vi "08Foot.vi"() -> ()   [LabVIEW 2015]
uses:
  <vilib>/Instr/_visa.llb/VISA Configure Serial Port (Serial Instr).vi
  <vilib>/Utility/file.llb/Read Delimited Spreadsheet (DBL).vi
  <vilib>/DAQmx/create/channels.llb/DAQmx Create Channel (DI-Digital Input).vi
  <vilib>/DAQmx/configure/timing.llb/DAQmx Timing (Sample Clock).vi
  <vilib>/Utility/file.llb/Write Delimited Spreadsheet (DBL).vi
  <resource>/objmgr/daqmx.rc
panel:
  in  "Tab Control":enum32{"Page 1", "Page 2"}(tab)
  out "NEXT MPH 2":dbl min=0.0 max=12.0 step=0.1 format="%.2f"
  out "MPH 2":dbl min=0.0 max=12.0 step=0.1 format="%.2f"
  out "NEXT DURATION":dbl format="%#.1f"
  out "Time Left":dbl format="%#.0f"
  out "ESTOP":bool
  in  "ESTOP RESUME":bool
  out "MPH READ":u8
  out "Foot":dbl
  out "ESTOP2":bool
  out "Report Location":path
  in  "TestScript":path=path "C:/LabVIEW VIs/TRMConsole/FootTime.txt"
  out "Waveform Graph":dbl[](graph)
  out "speed":dbl[](array[numeric])
  out "time":dbl[](array[numeric])
  out "dwell":dbl[](array[numeric])
  out "step":i32
  out "arraysize":i32
  out "x-y":u32
  out "appended path":path
  out "stopping":bool
  out "String":string
  in  "stop":bool
  in  "Serial Port":refnum<visa-resource-name>="COM8"
  in  "lines":tag="DAQMod1/port0"
  out "Enum":T1(ring)
  out "NEXT MPH":dbl min=0.0 max=12.0 step=0.1 format="%.1f"
  out "MPH":dbl min=0.0 max=12.0 step=0.1 format="%.1f"
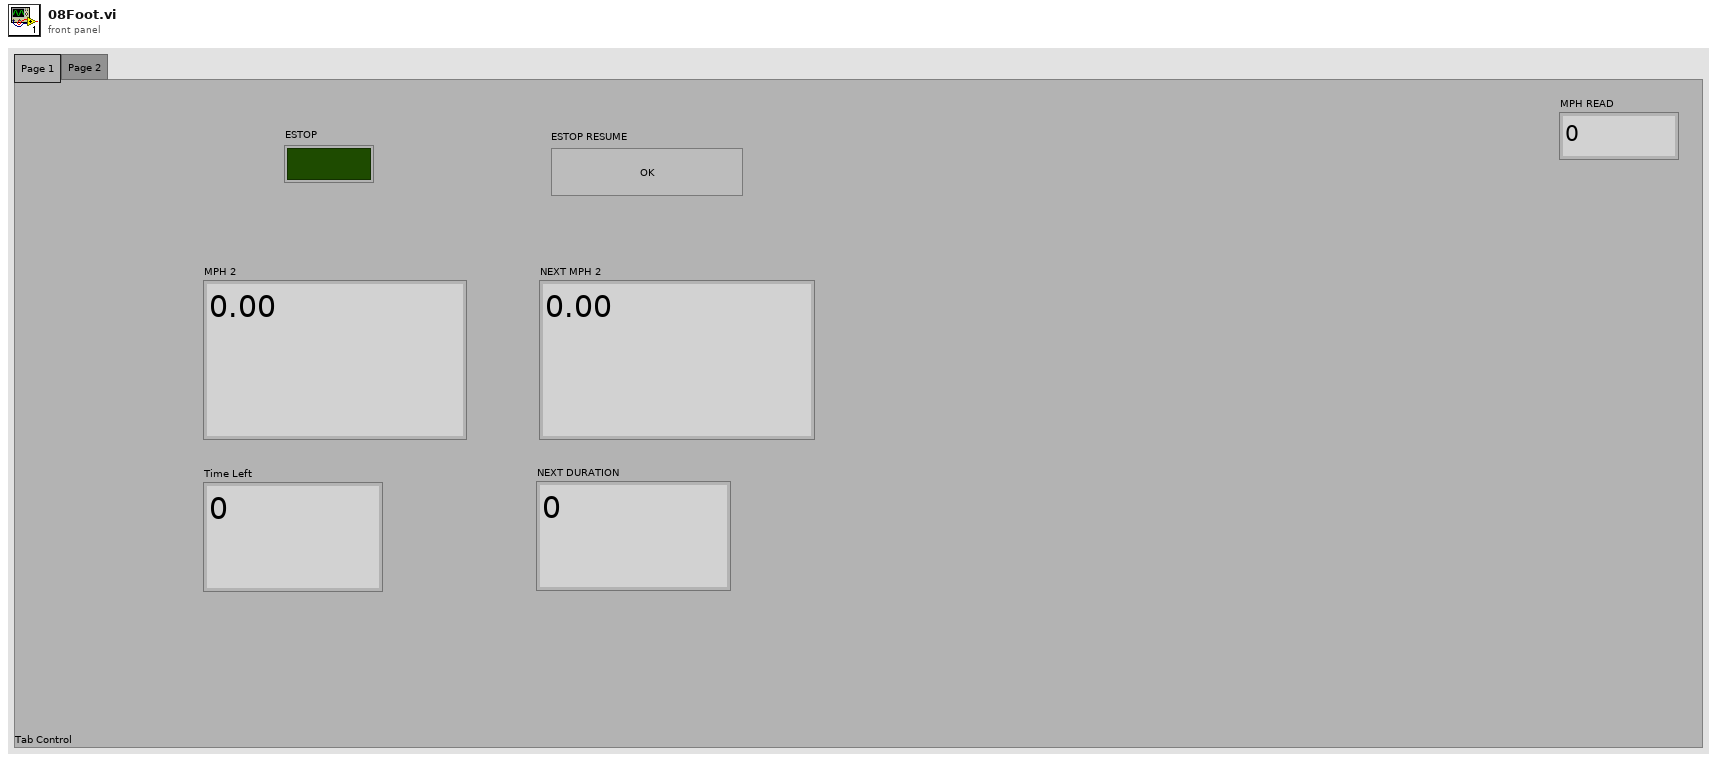
[diagram p1: front panel]
types:
  T1 = enum16{"Initialize", "SetMPH", "GetData", "CheckTiming", "CompressWave", "StartDAQ", "StopDAQ", "Dwell", "WaitforMPH", "ESTOP Wait", "ESTOP Resume"}
  T2 = enum16{"Initialize", "SetMPH", "GetData", "CheckTiming", "CompressWave", "StartDAQ", "StopDAQ", "Dwell", "WaitforMPH"}
  T3 = enum16{"Initialize", "SetMPH", "GetData", "CheckTiming", "CompressWave", "StartDAQ"}
  T4 = enum16{"Initialize", "SetMPH", "GetData", "CheckTiming", "CompressWave"}
  T5 = enum16{"Initialize", "SetMPH", "GetData", "CheckTiming", "CompressWave", "StartDAQ", "StopDAQ"}
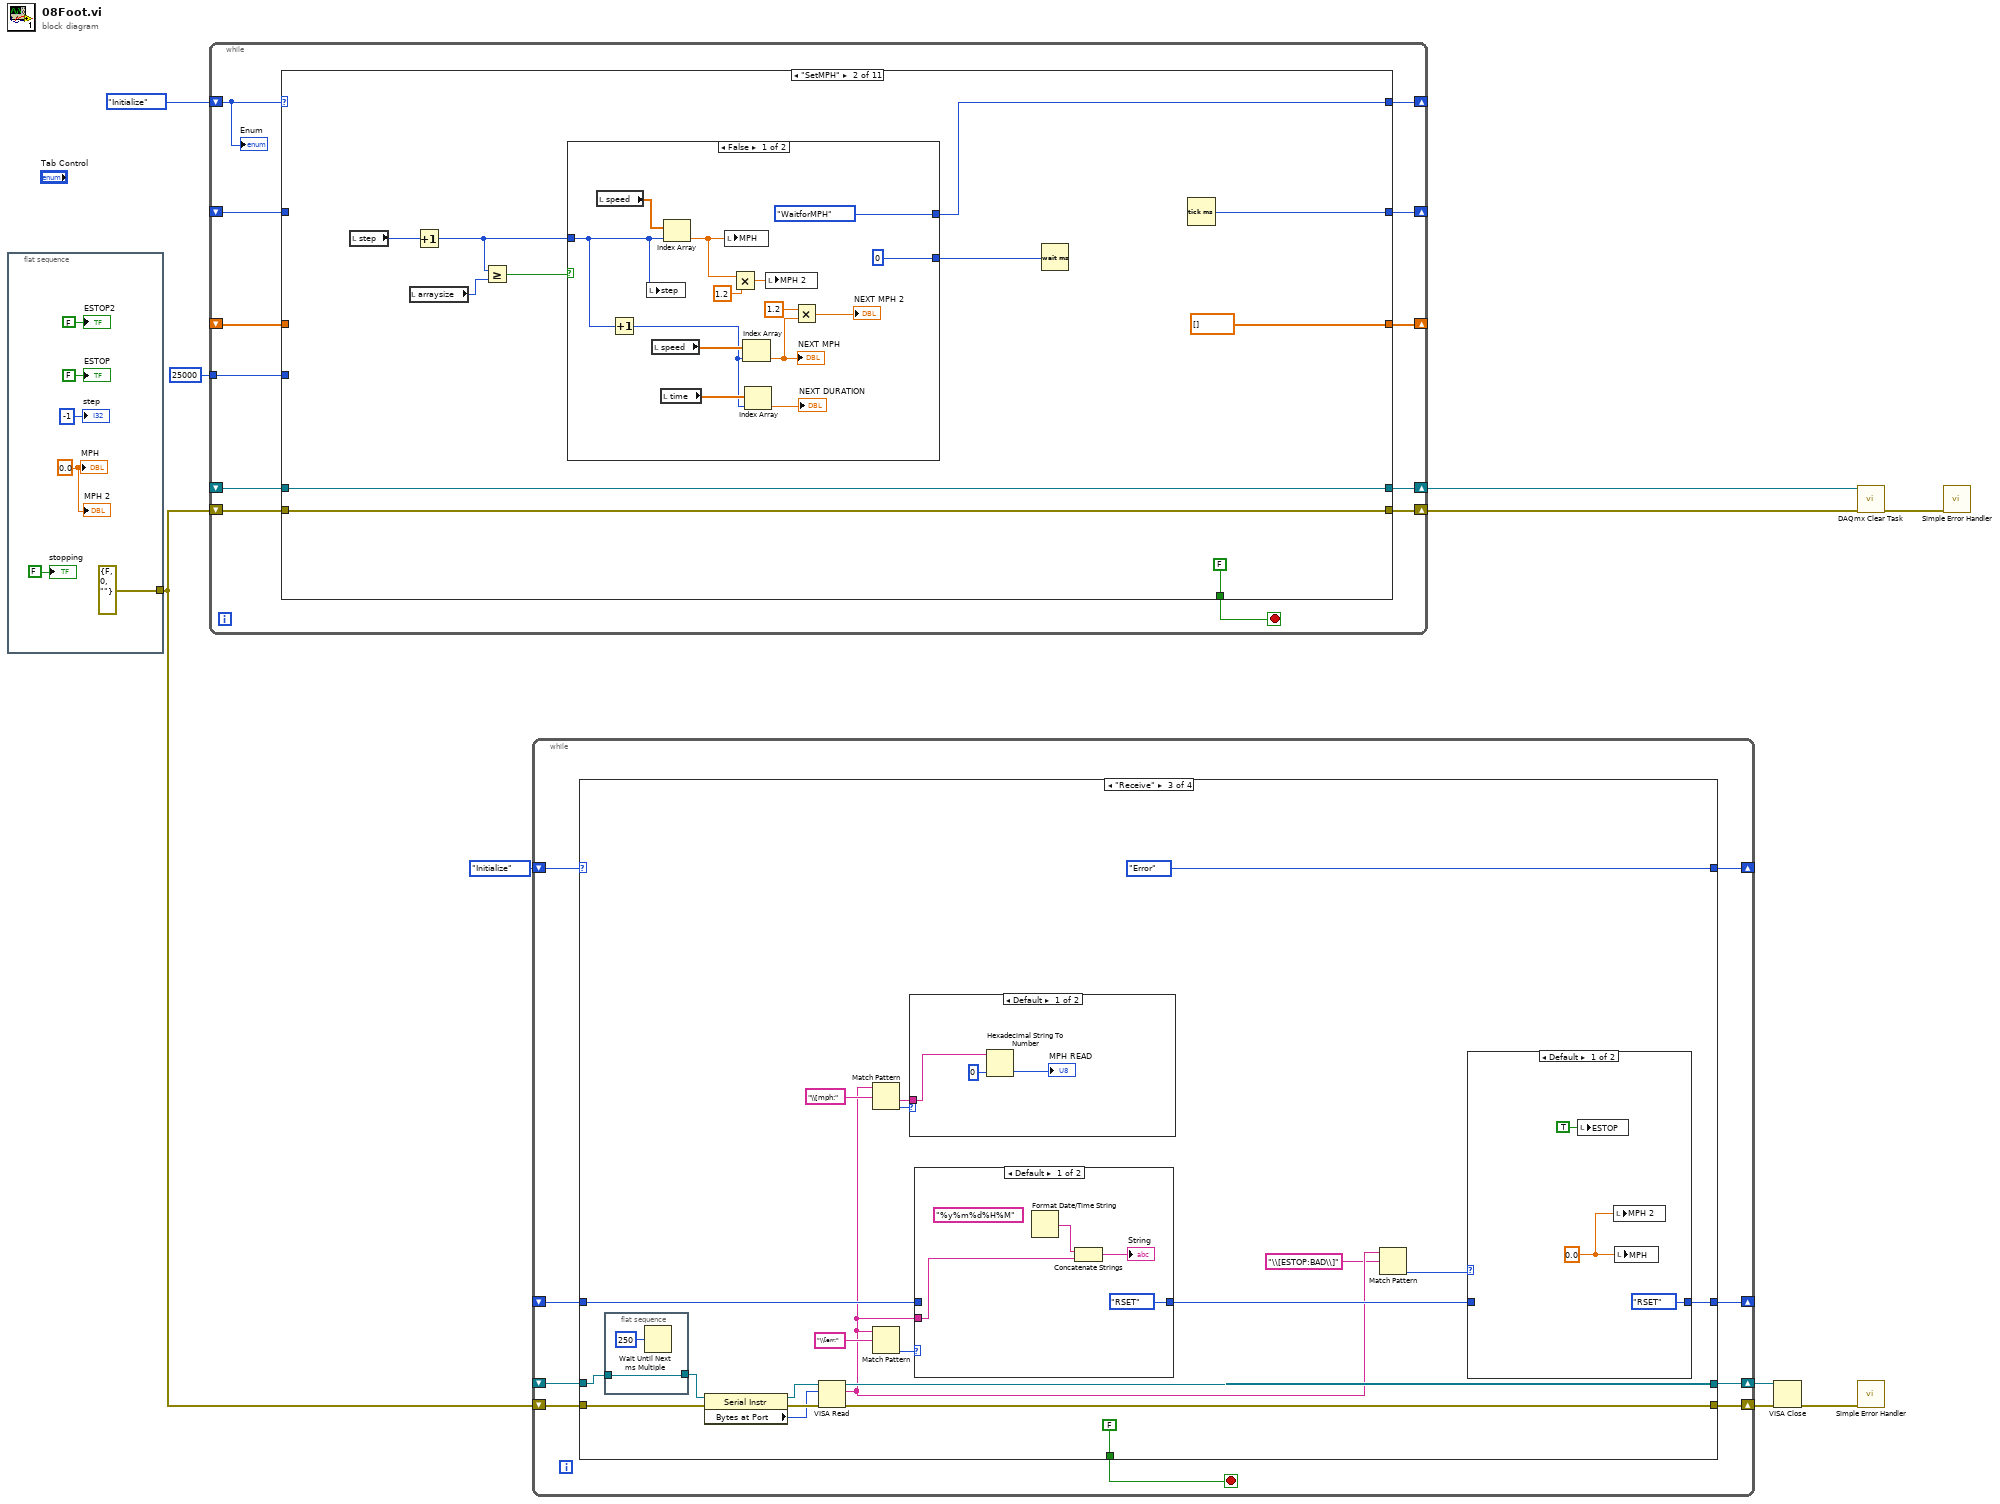
[diagram p0: block diagram]
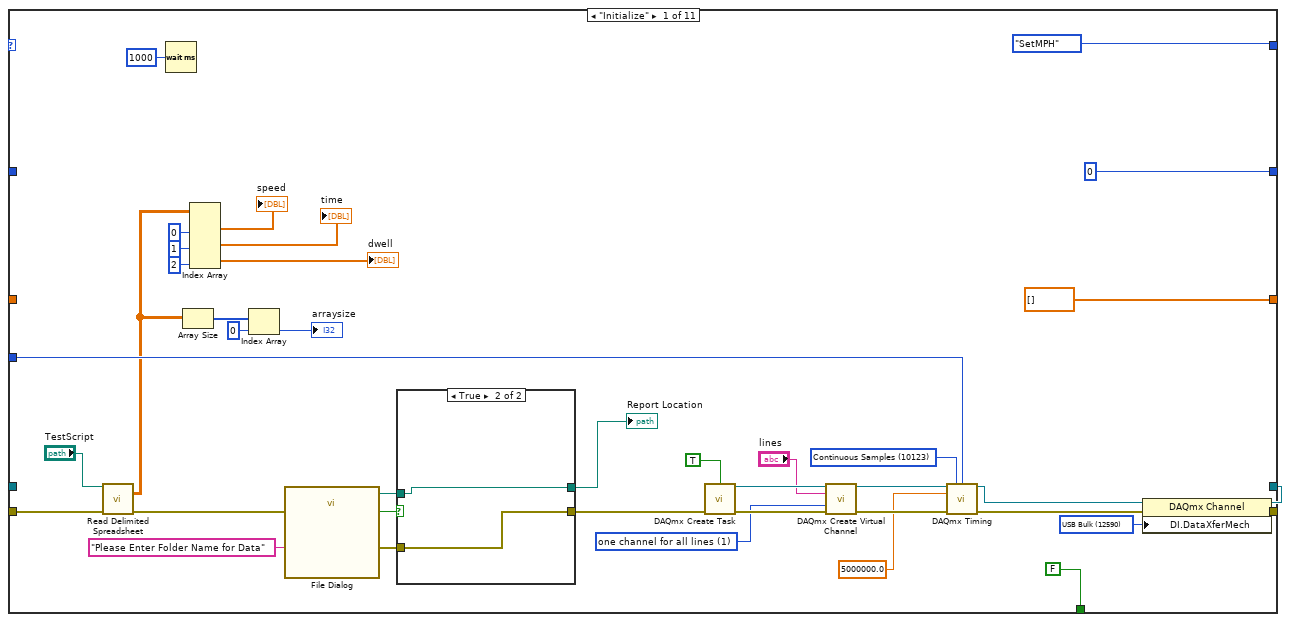
[diagram p2: hidden frame]
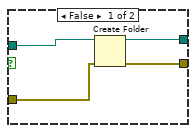
[diagram p3: hidden frame]
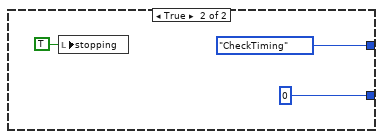
[diagram p4: hidden frame]
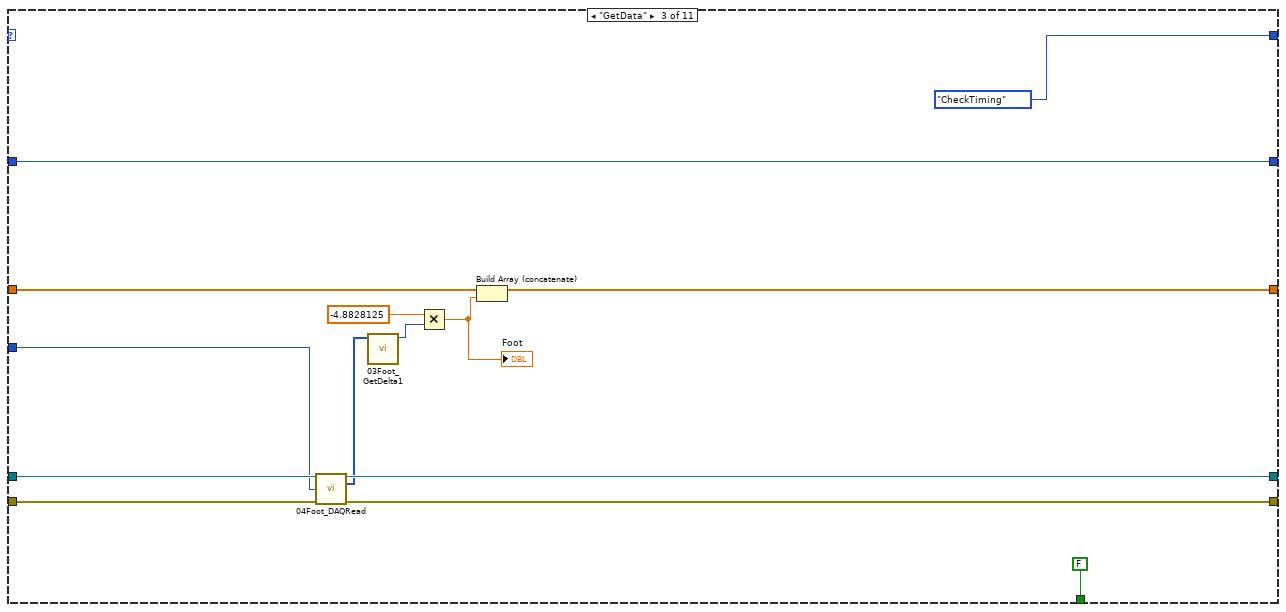
[diagram p5: hidden frame]
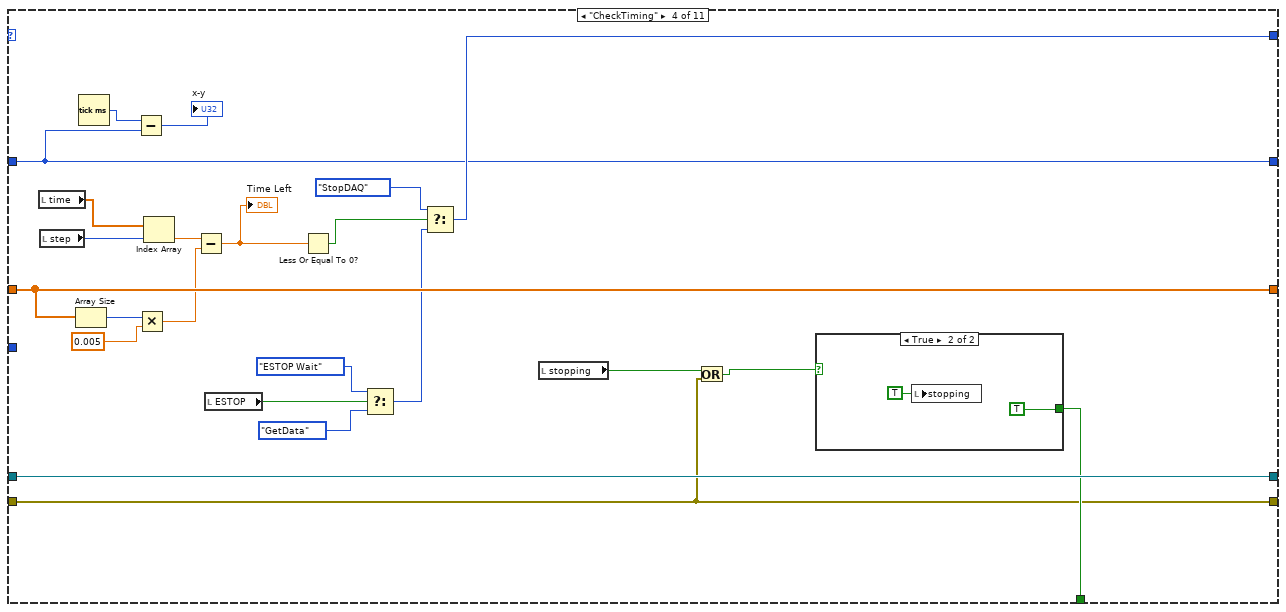
[diagram p6: hidden frame]
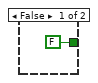
[diagram p7: hidden frame]
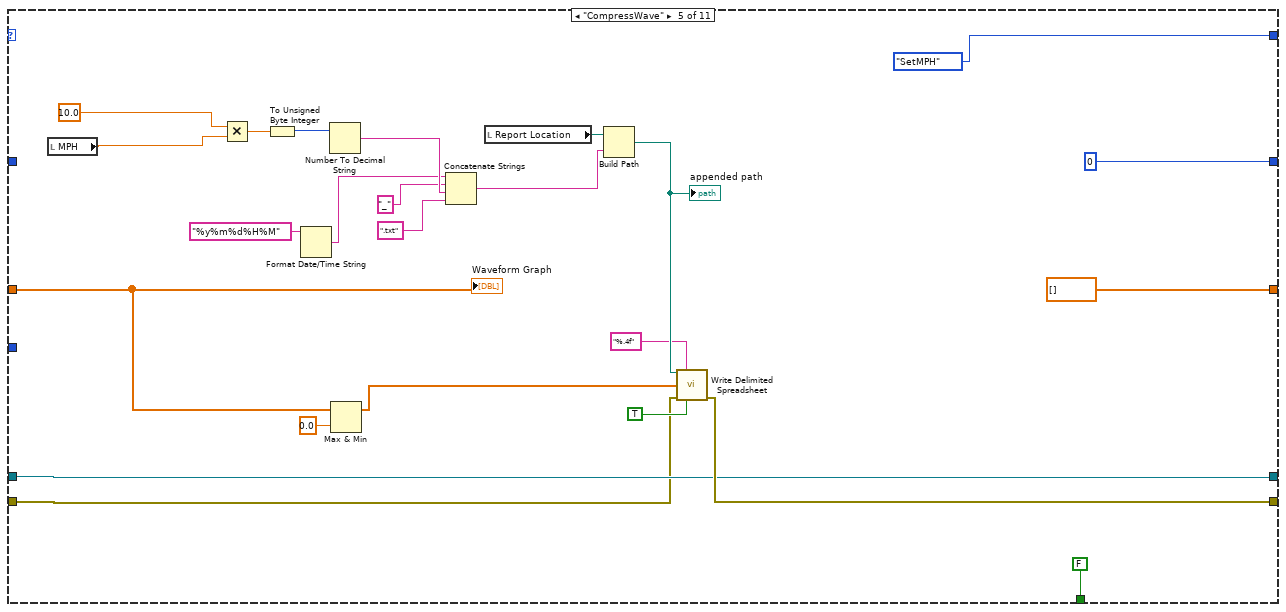
[diagram p8: hidden frame]
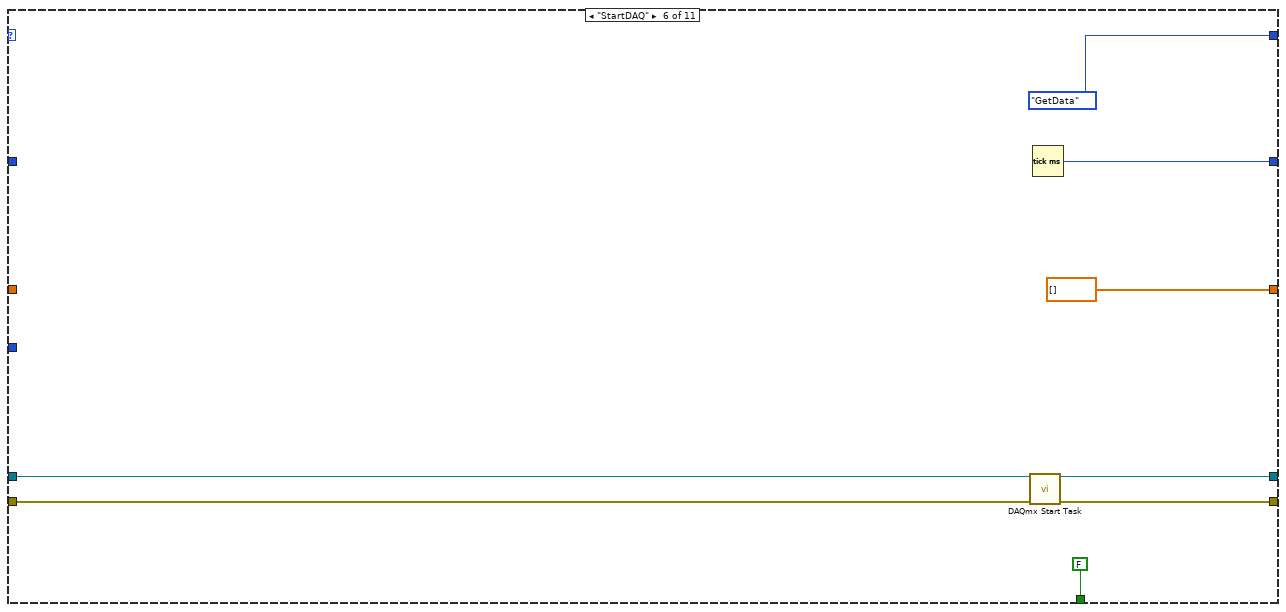
[diagram p9: hidden frame]
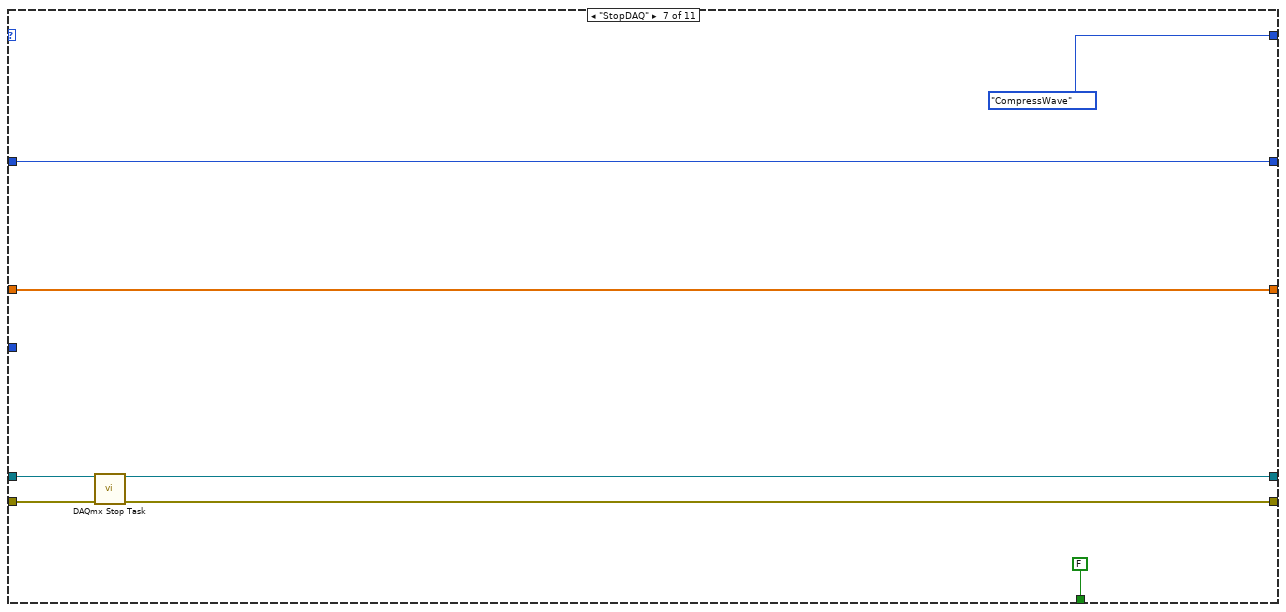
[diagram p10: hidden frame]
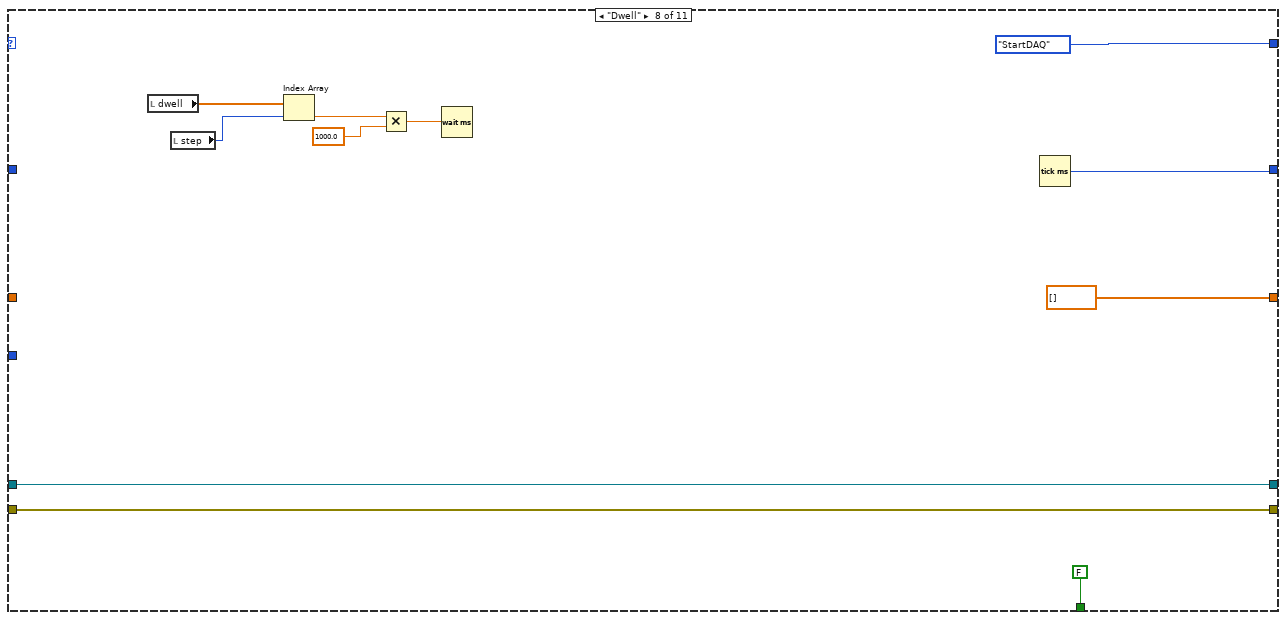
[diagram p11: hidden frame]
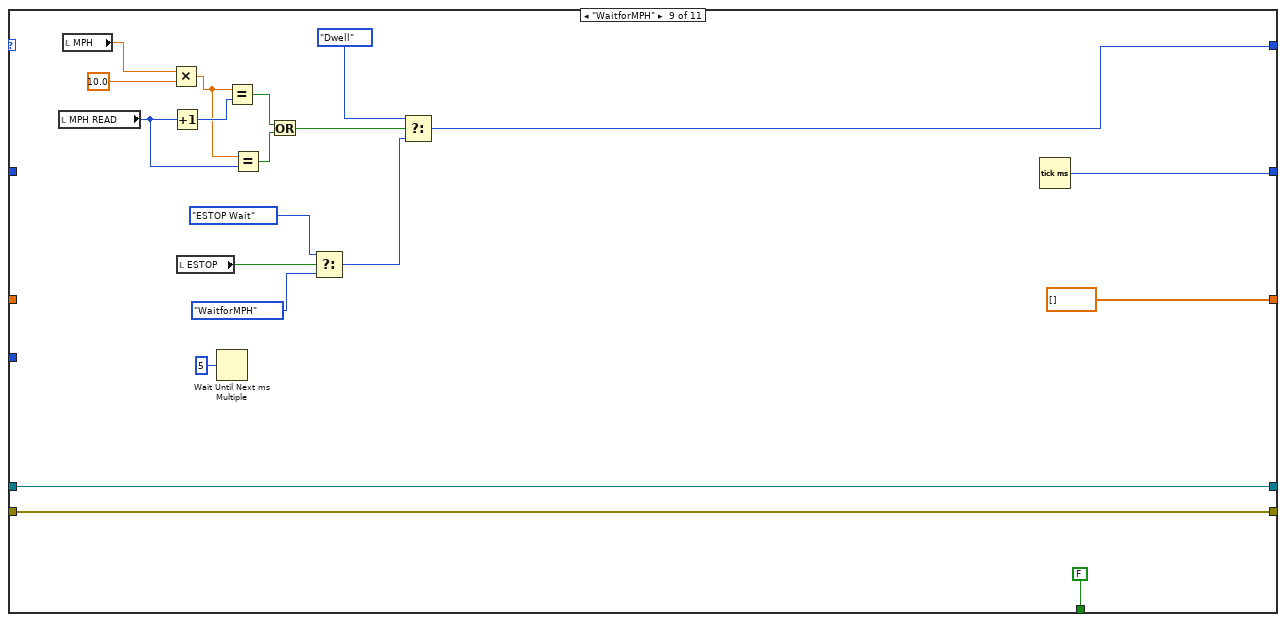
[diagram p12: hidden frame]
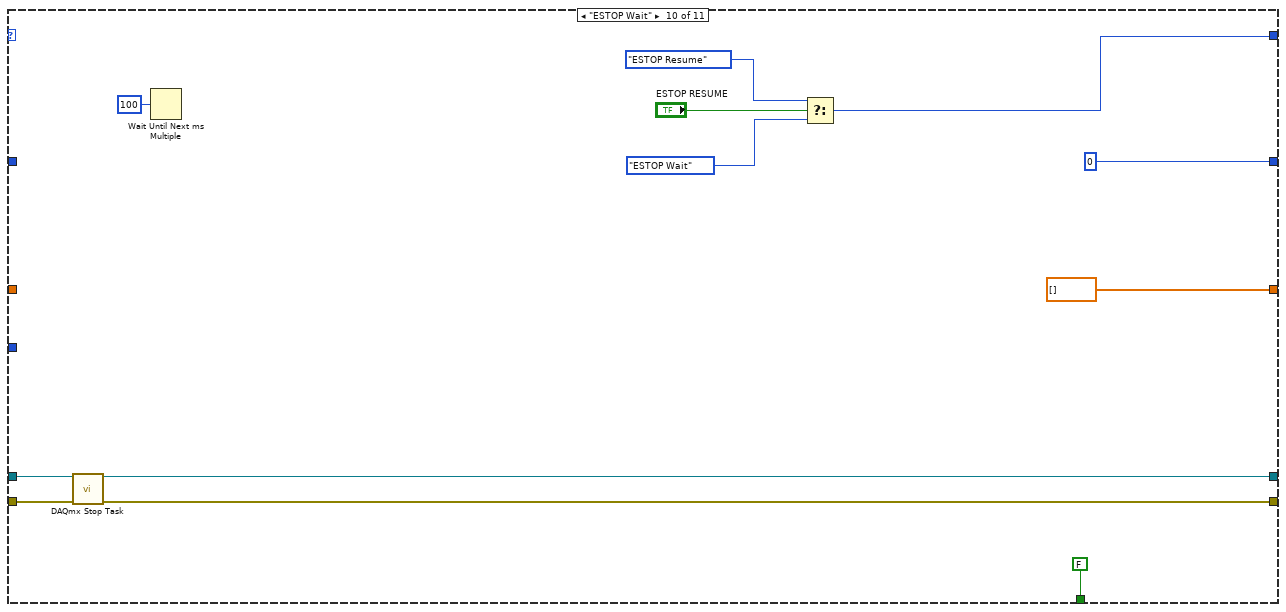
[diagram p13: hidden frame]
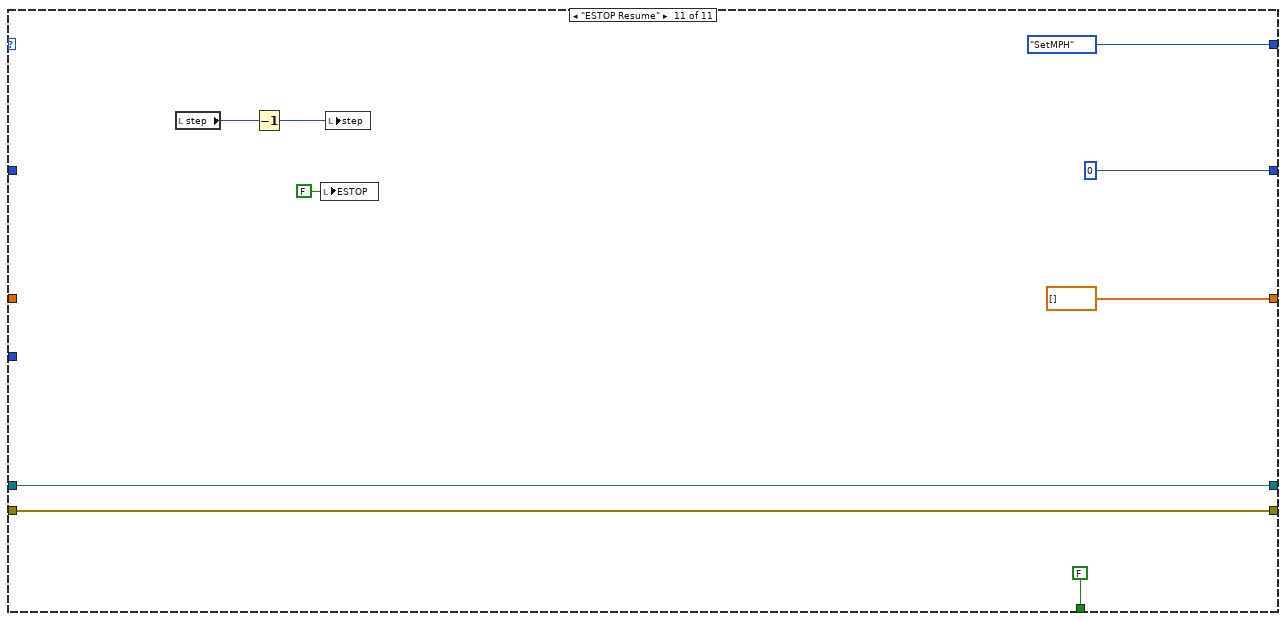
[diagram p14: hidden frame]
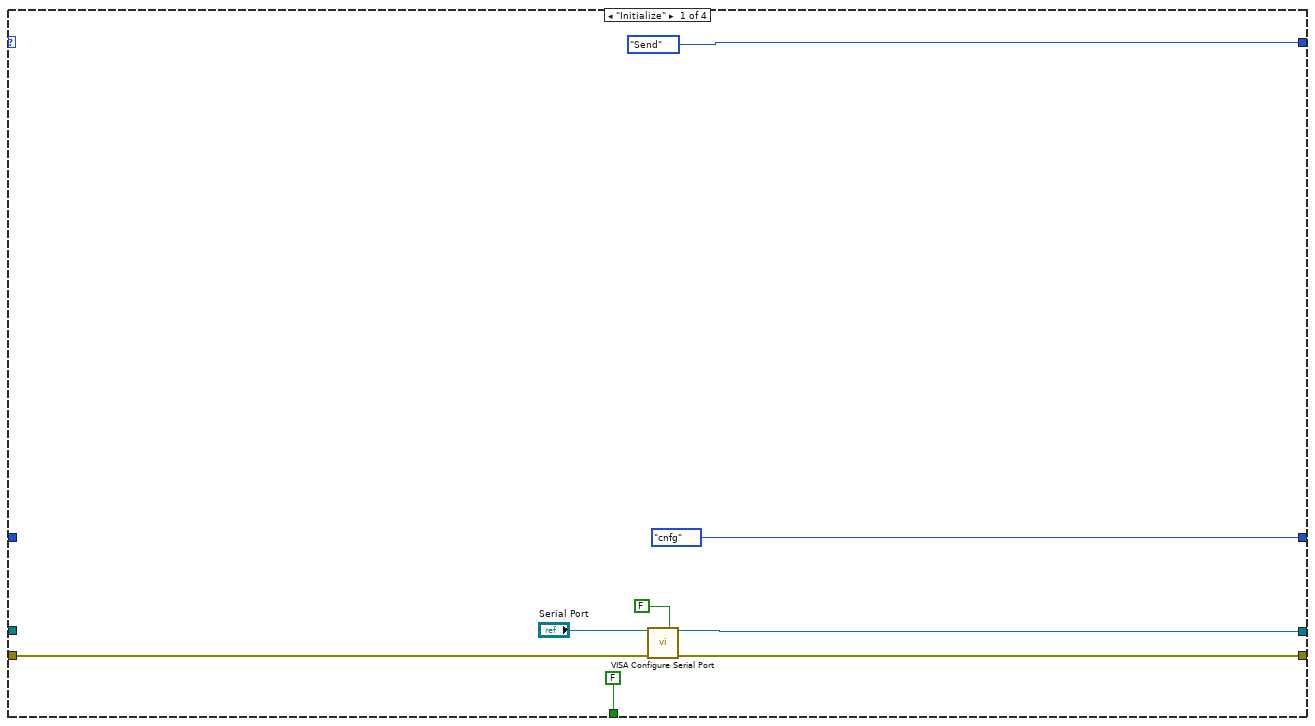
[diagram p15: hidden frame]
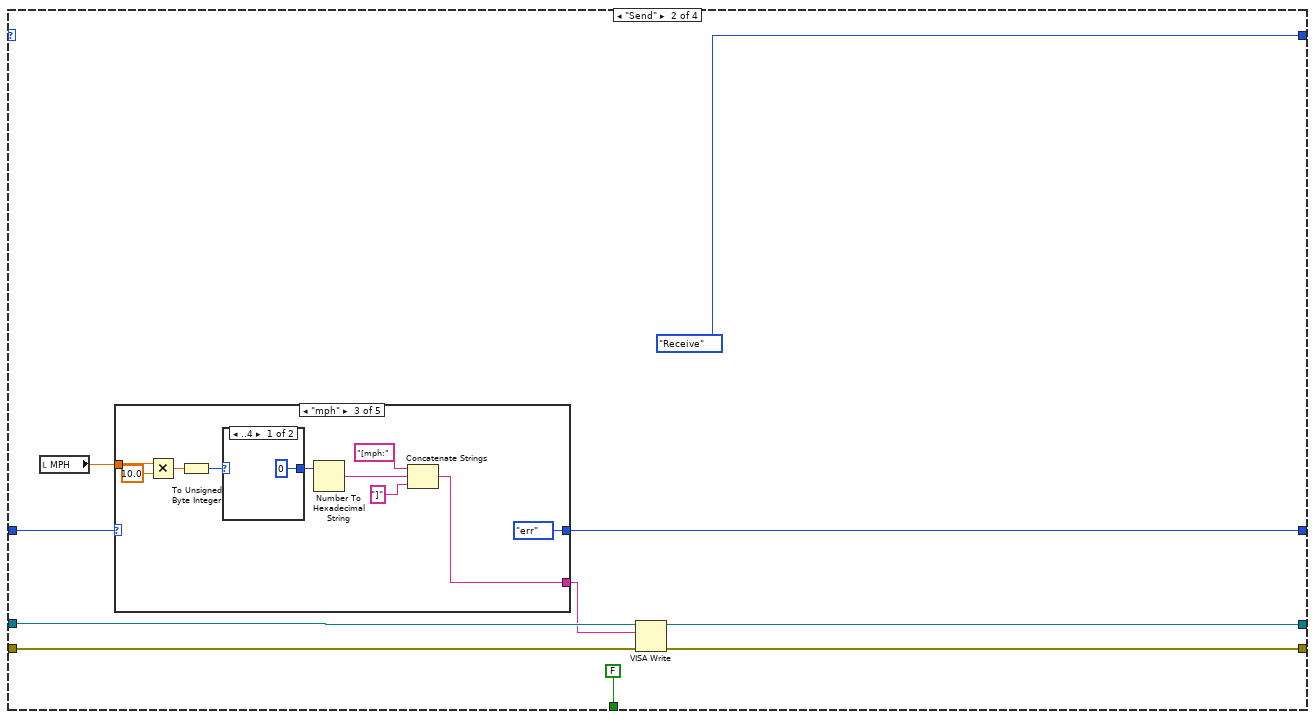
[diagram p16: hidden frame]
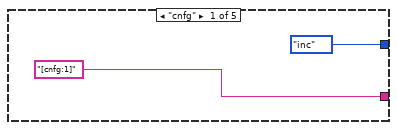
[diagram p17: hidden frame]
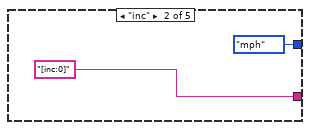
[diagram p18: hidden frame]
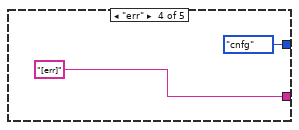
[diagram p20: hidden frame]
diagram:
  n1 = flat-sequence {
    tunnel: [errorcluster {"status"=FALSE, "code"=0, "source"=""} ("error constant")] -> w2
    frame #0 {
      w11 = 0.0 ("MPH")
      "stopping" <- FALSE ("stopping")
      "MPH" <- w11
      "step" <- -1 ("step")
      "ESTOP" <- FALSE ("ESTOP")
      "ESTOP2" <- FALSE ("ESTOP2")
      "MPH 2" <- w11
    }
  }
  n2 = while {
    shift-right: [w28] -> _
    shift-left: T1."Initialize" -> [w17]
    shift-right: [w26] -> w4
    shift-left: _ -> [w24]
    shift-right: [w25] -> w5
    shift-left: w2 -> [w23]
    shift-right: [w22] -> _
    shift-left: _ -> [w21]
    tunnel: 25000 ("samples per channel") -> [w20]
    shift-right: [w19] -> _
    shift-left: _ -> [w18]
    stop <- w27 stop-if-true
    n3 = case shown="\"SetMPH\"" w17 {
      tunnel: [T1."SetMPH" w78 T4."CheckTiming" w132 T1."SetMPH" T3."GetData" T5."CompressWave" T2."StartDAQ" w204 w219 T1."SetMPH" ("f")] -> w28
      tunnel: [FALSE FALSE FALSE w136 FALSE FALSE FALSE FALSE FALSE FALSE FALSE] -> w27
      tunnel: [w31 w81 w108 w138 w149 w168 w177 w190 w210 w214 w227] -> w26
      tunnel: [w30 w80 w107 w133 w162 w169 w176 w189 w209 w213 w228] -> w25
      tunnel: w24 -> [_ w81 w110 w138 w149 w167 w179 w190 w210 w216 w227]
      tunnel: w23 -> [w58 w80 w109 w133 w148 w166 w178 w189 w209 w215 w228]
      tunnel: [u32 0 w79 w114 w116 u32 0 w172 w174 w192 w212 u32 0 ("millisecond timer value") u32 0 ("millisecond timer value")] -> w22
      tunnel: w21 -> [_ _ w114 w116 _ _ w174 _ _ _ _]
      tunnel: w20 -> [w55 _ w106 _ _ _ _ _ _ _ _]
      tunnel: [dbl[] [] dbl[] [] w113 w131 dbl[] [] dbl[] [] w180 dbl[] [] dbl[] [] dbl[] [] dbl[] []] -> w19
      tunnel: w18 -> [_ _ w112 w131 w143 _ w180 _ _ _ _]
      frame "Initialize" {
        w29 = 12590 items=["DMA"=10054, "Interrupts"=10204, "Programmed I/O"=10264, "USB Bulk"=12590] ("DI.DataXferMech")
        w54 = 10123 items=["Finite Samples"=10178, "Continuous Samples"=10123, "Hardware Timed Single Point"=12522] ("sample mode")
        w65 = 1 items=["one channel for each line", "one channel for all lines"] ("line grouping")
        n4 = call-poly <vilib>:"Read Delimited Spreadsheet.vi"("file path (dialog if empty)"="TestScript", "error in (no error)"=w58) -> ("all rows"=w43:dbl[][], "error out"=w41:errorcluster)  [unwired: 8 in, 4 out]
        n5 = Wait (ms)(milliseconds to wait=u32 1000) -> ()  [unwired: 1 out]
        n6 = Array Size(array=w43) -> (size(s)=w46:i32[])
        n7 = Index Array(array=w43, index (col) #1=0 ("disabled index (col)"), index (col) #2=1 ("index (col)"), index (col) #3=2 ("index (col)")) -> (element #1=→"speed":dbl[], element #2=→"time":dbl[], element #3=→"dwell":dbl[])  [unwired: 3 in]
        n8 = Index Array(array=w46, index=0) -> (element=→"arraysize":i32)
        n9 = call "File Dialog"("prompt"="Please Enter Folder Name for Data", "error in"=w41) -> ("selected path"=w37:path, "exists"=w39:bool, "error out"=w38:errorcluster)  [unwired: 10 in, 1 out]
        n10 = case shown="True" w39 {
          tunnel: w38 -> [w71 w72]
          tunnel: w37 -> [w70 w73]
          tunnel: [w69 w72] -> w36
          tunnel: [w68 w73] -> w35
          frame False {
            n11 = Create Folder(path (use dialog)=w70, error in=w71) -> (created path=w68:path, error out=w69:errorcluster)  [unwired: 1 in, 1 out]
          }
          frame True {
          }
        }
        "Report Location" <- w35
        n12 = call <vilib>:"DAQmx Create Task.vi"("auto cleanup"=TRUE, "error in"=w36) -> ("task out"=w67:refnum<k21>, "error out"=w66:errorcluster)  [unwired: 12 in]
        n13 = call-poly <vilib>:"DAQmx Create Virtual Channel.vi"("task in"=w67, "lines"="lines", "line grouping"=w65, "error in"=w66) -> ("task out"=w56:refnum<k21>, "error out"=w57:errorcluster)  [unwired: 10 in]
        n14 = call-poly <vilib>:"DAQmx Timing.vi"("task/channels in"=w56, "sample mode"=w54, "samples per channel"=w55, "rate"=5000000.0, "error in"=w57) -> ("task out"=w33:refnum<k21>, "error out"=w32:errorcluster)  [unwired: 9 in]
        n15 = property class="DAQmx Channel"(reference=w33, error in=w32, "DI.DataXferMech"=w29) -> (reference out=w31:refnum<k21>, error out=w30:errorcluster)
      }
      frame "SetMPH" {
        n16 = local read "step"() -> (w75:i32)
        n17 = local read "arraysize"() -> (w77:i32)
        n18 = Increment(x=w75) -> (x+1=w74:i32)
        n19 = Greater Or Equal?(x=w74, y=w77) -> (x >= y?=w76:bool)
        n20 = case shown="False" w76 {
          tunnel: [u32 0 ("milliseconds to wait") u32 0 ("milliseconds to wait")] -> w83
          tunnel: [T2."WaitforMPH" T3."CheckTiming"] -> w78
          tunnel: w74 -> [w95 _]
          frame False {
            n21 = local read "speed"() -> (w97:dbl[])
            n22 = Increment(x=w95) -> (x+1=w91:i32)
            n23 = local write "step"(w95) -> ()
            n24 = local read "speed"() -> (w94:dbl[])
            n25 = local read "time"() -> (w92:dbl[])
            n26 = Index Array(array=w97, index=w95) -> (element=w90:dbl)
            n27 = local write "MPH"(w90) -> ()
            n28 = Multiply(x=w90, y=1.2 ("element")) -> (x*y=w88:dbl)
            n29 = Index Array(array=w94, index=w91) -> (element=w87:dbl)
            "NEXT MPH" <- w87
            n30 = Index Array(array=w92, index=w91) -> (element=→"NEXT DURATION":dbl)
            n31 = local write "MPH 2"(w88) -> ()
            n32 = Multiply(x=1.2, y=w87) -> (x*y=→"NEXT MPH 2":dbl)
          }
          frame True {
            n33 = local write "stopping"(TRUE ("stopping")) -> ()
          }
        }
        n34 = Wait (ms)(milliseconds to wait=w83) -> ()  [unwired: 1 out]
        n35 = Tick Count (ms)() -> (millisecond timer value=w79:u32)
      }
      frame "GetData" {
        n36 = call "04Foot_DAQRead.vi"("task/channels in"=w110, "number of samples per channel"=w106, "error in"=w109) -> ("task out"=w108:refnum<k21>, "data"=w105:u8[], "error out"=w107:errorcluster)  [unwired: 10 in]
        n37 = call "03Foot_GetDelta1.vi"("Array"=w105) -> ("Wave1 Data"=w104:i32)  [unwired: 10 in]
        n38 = Multiply(x=-4.8828125, y=w104) -> (x*y=w102:dbl)
        "Foot" <- w102
        n39 = Build Array (concatenate)(w112, w102) -> (w113:dbl[])
      }
      frame "CheckTiming" {
        n40 = local read "time"() -> (w128:dbl[])
        n41 = local read "step"() -> (w127:i32)
        n42 = Array Size(array=w131) -> (size(s)=w130:i32)
        n43 = Tick Count (ms)() -> (millisecond timer value=w117:u32)
        n44 = Subtract(x=w117, y=w116) -> (x-y=→"x-y":u32)
        n45 = Multiply(x=w130, y=0.005) -> (x*y=w120:dbl)
        n46 = Index Array(array=w128, index=w127) -> (element=w121:dbl)
        n47 = Subtract(x=w121, y=w120) -> (x-y=w119:dbl)
        "Time Left" <- w119
        n48 = local read "ESTOP"() -> (w124:bool)
        n49 = Less Or Equal To 0?(x=w119) -> (x <= 0?=w118:bool)
        n50 = Select(t=T1."ESTOP Wait", s=w124, f=T1."GetData") -> (s? t:f=w122:T1)
        n51 = Select(t=T1."StopDAQ", s=w118, f=w122) -> (s? t:f=w132:T1)
        n52 = local read "stopping"() -> (w135:bool)
        n53 = Or(x=w135, y=w133) -> (x .or. y?=w134:bool)
        n54 = case shown="True" w134 {
          tunnel: [FALSE TRUE] -> w136
          frame False {
          }
          frame True {
            n55 = local write "stopping"(TRUE ("stopping")) -> ()
          }
        }
      }
      frame "CompressWave" {
        n56 = local read "MPH"() -> (w152:dbl)
        n57 = Multiply(x=10.0, y=w152) -> (x*y=w155:dbl)
        n58 = To Unsigned Byte Integer(number=w155) -> (unsigned 8bit integer=w154:u8)
        n59 = Format Date/Time String(time format string (%c)="%y%m%d%H%M") -> (date/time string=w144:string)  [unwired: 2 in]
        n60 = Number To Decimal String(number=w154) -> (decimal integer string=w153:string)  [unwired: 1 in]
        n61 = Max & Min(x=w143, y=0.0) -> (max(x,y)=w150:dbl[])  [unwired: 1 out]
        n62 = Concatenate Strings(w144, "_" ("string"), w153, ".txt" ("string")) -> (w158:string)
        n63 = local read "Report Location"() -> (w147:path)
        n64 = Build Path(base path=w147, name or relative path=w158) -> (appended path=w157:path)
        "appended path" <- w157
        n65 = call-poly <vilib>:"Write Delimited Spreadsheet.vi"("file path (dialog if empty)"=w157, "format (%.3f)"="%.4f", "1D data"=w150, "error in (no error)"=w148, "transpose? (F)"=TRUE) -> ("error out"=w162:errorcluster)  [unwired: 9 in, 1 out]
        "Waveform Graph" <- w143
      }
      frame "StartDAQ" {
        n66 = call <vilib>:"DAQmx Start Task.vi"("task/channels in"=w167, "error in"=w166) -> ("task out"=w168:refnum<k21>, "error out"=w169:errorcluster)  [unwired: 12 in]
        n67 = Tick Count (ms)() -> (millisecond timer value=w172:u32)
      }
      frame "StopDAQ" {
        n68 = call <vilib>:"DAQmx Stop Task.vi"("task/channels in"=w179, "error in"=w178) -> ("task out"=w177:refnum<k21>, "error out"=w176:errorcluster)  [unwired: 12 in]
      }
      frame "Dwell" {
        n69 = local read "dwell"() -> (w187:dbl[])
        n70 = local read "step"() -> (w186:i32)
        n71 = Index Array(array=w187, index=w186) -> (element=w185:dbl)
        n72 = Multiply(x=w185, y=1000.0) -> (x*y=w183:dbl)
        n73 = Wait (ms)(milliseconds to wait=w183) -> ()  [unwired: 1 out]
        n74 = Tick Count (ms)() -> (millisecond timer value=w192:u32)
      }
      frame "WaitforMPH" {
        n75 = local read "MPH READ"() -> (w196:u8)
        n76 = local read "MPH"() -> (w207:dbl)
        n77 = Multiply(x=w207, y=10.0) -> (x*y=w197:dbl)
        n78 = Increment(x=w196) -> (x+1=w205:u8)
        n79 = local read "ESTOP"() -> (w202:bool)
        n80 = Wait Until Next ms Multiple(millisecond multiple=u32 5) -> ()  [unwired: 1 out]
        n81 = Equal?(x=w197, y=w205) -> (x = y?=w194:bool)
        n82 = Equal?(x=w197, y=w196) -> (x = y?=w195:bool)
        n83 = Or(x=w194, y=w195) -> (x .or. y?=w193:bool)
        n84 = Select(t=T1."ESTOP Wait", s=w202, f=T1."WaitforMPH") -> (s? t:f=w199:T1)
        n85 = Select(t=T1."Dwell", s=w193, f=w199) -> (s? t:f=w204:T1)
        n86 = Tick Count (ms)() -> (millisecond timer value=w212:u32)
      }
      frame "ESTOP Wait" {
        n87 = call <vilib>:"DAQmx Stop Task.vi"("task/channels in"=w216, "error in"=w215) -> ("task out"=w214:refnum<k21>, "error out"=w213:errorcluster)  [unwired: 12 in]
        n88 = Wait Until Next ms Multiple(millisecond multiple=u32 100) -> ()  [unwired: 1 out]
        n89 = Select(t=T1."ESTOP Resume", s="ESTOP RESUME", f=T1."ESTOP Wait") -> (s? t:f=w219:T1)
      }
      frame "ESTOP Resume" {
        n90 = local read "step"() -> (w233:i32)
        n91 = Decrement(x=w233) -> (x-1=w232:i32)
        n92 = local write "ESTOP"(FALSE ("ESTOP")) -> ()
        n93 = local write "step"(w232) -> ()
      }
    }
    "Enum" <- w17
  }
  n94 = while {
    shift-right: [w238] -> w8
    shift-left: w2 -> [w242]
    shift-right: [w239] -> w9
    shift-left: _ -> [w241]
    shift-right: [w237] -> _
    shift-left: enum16{"Initialize", "Send", "Receive", "Error"}."Initialize" -> [w240]
    shift-right: [w236] -> _
    shift-left: _ -> [w235]
    stop <- w234 stop-if-true
    n95 = case shown="\"Receive\"" w240 {
      tunnel: w242 -> [w246 w258 w297 w317]
      tunnel: w241 -> [_ w257 w296 w321]
      tunnel: [w248 w260 w295 w321] -> w239
      tunnel: [w247 w259 w289 w317] -> w238
      tunnel: [enum16{"Initialize", "Send", "Receive", "Error"}."Send" enum16{"Initialize", "Send", "Receive", "Error"}."Receive" enum16{"Initialize", "Send", "Receive", "Error"}."Error" enum16{"Initialize", "Send", "Receive", "Error"}."Send"] -> w237
      tunnel: [enum16{"cnfg", "inc", "mph", "err", "RSET"}."cnfg" w254 w283 w322] -> w236
      tunnel: w235 -> [_ w255 w290 w322]
      tunnel: [FALSE FALSE FALSE w316] -> w234
      frame "Initialize" {
        n96 = call-poly "VISA Configure Serial Port"("VISA resource name"="Serial Port", "Enable Termination\nChar (T)"=FALSE ("Enable Termination\nChar (T)"), "error in (no error)"=w246) -> ("VISA resource name out"=w248:refnum<visa-resource-name>, "error out"=w247:errorcluster)  [unwired: 11 in]
      }
      frame "Send" {
        n97 = local read "MPH"() -> (w251:dbl)
        n98 = case shown="\"mph\"" w255 {
          tunnel: ["[cnfg:1]" "[inc:0]" w265 "[err]" "[RSET]"] -> w256
          tunnel: w251 -> [_ _ w274 _ _]
          tunnel: [enum16{"cnfg", "inc", "mph", "err", "RSET"}."inc" enum16{"cnfg", "inc", "mph", "err", "RSET"}."mph" enum16{"cnfg", "inc", "mph", "err", "RSET"}."err" enum16{"cnfg", "inc", "mph", "err", "RSET"}."cnfg" enum16{"cnfg", "inc", "mph", "err", "RSET"}."cnfg"] -> w254
          frame "cnfg" {
          }
          frame "inc" {
          }
          frame "mph" {
            n99 = Multiply(x=w274, y=10.0) -> (x*y=w268:dbl)
            n100 = To Unsigned Byte Integer(number=w268) -> (unsigned 8bit integer=w267:u8)
            n101 = case shown="..4" w267 {
              selector: w267 -> [_ w276]
              tunnel: [u8 0 w276] -> w266
              frame ..4 {
              }
              frame 5.. {
              }
            }
            n102 = Number To Hexadecimal String(2:w266) -> (0:w271:string)  [unwired: 1 in]
            n103 = Concatenate Strings("[mph:" ("string"), w271, "]" ("string")) -> (w265:string)
          }
          frame "err" {
          }
          frame "RSET" {
          }
        }
        n104 = VISA Write(VISA resource name=w257, write buffer=w256, error in (no error)=w258) -> (VISA resource name out=w260:refnum<visa-resource-name>, error out=w259:errorcluster)  [unwired: 1 out]
      }
      frame "Receive" {
        n105 = flat-sequence {
          tunnel: w296 -> [w314]
          tunnel: [w314] -> w301
          frame #0 {
            n106 = Wait Until Next ms Multiple(millisecond multiple=u32 250) -> ()  [unwired: 1 out]
          }
        }
        n107 = property class="Serial Instr"(reference=w301, error in=w297) -> (reference out=w299:refnum<visa-resource-name>, error out=w300:errorcluster, "Bytes at Port"=w298:u32)
        n108 = VISA Read(VISA resource name=w299, byte count=w298, error in (no error)=w300) -> (VISA resource name out=w295:refnum<visa-resource-name>, read buffer=w284:string, error out=w289:errorcluster)  [unwired: 1 out]
        n109 = Match Pattern(string=w284, regular expression="\\[mph:") -> (after substring=w286:string, offset past match=w287:i32)  [unwired: 1 in, 2 out]
        n110 = Match Pattern(string=w284, regular expression="\\[err:") -> (offset past match=w291:i32)  [unwired: 1 in, 3 out]
        n111 = case shown="Default" w287 {
          tunnel: w286 -> [w308 _]
          frame Default {
            n112 = Hexadecimal String To Number(string=w308, default (0uL)=u8 0 ("default (0 I32)")) -> (number=→"MPH READ":u8)  [unwired: 1 in, 1 out]
          }
          frame -1 {
          }
        }
        n113 = case shown="Default" w291 {
          tunnel: [enum16{"cnfg", "inc", "mph", "err", "RSET"}."RSET" w313] -> w285
          tunnel: w290 -> [_ w313]
          tunnel: w284 -> [w309 _]
          frame Default {
            (unwired) "%y%m%d%H%M" ("time format string (%c)")
            n114 = Format Date/Time String() -> (date/time string=w310:string)  [unwired: 3 in]
            n115 = Concatenate Strings(w310, w309) -> (→"String":string)
          }
          frame -1 {
          }
        }
        n116 = Match Pattern(string=w284, regular expression="\\[ESTOP:BAD\\]") -> (offset past match=w282:i32)  [unwired: 1 in, 3 out]
        n117 = case shown="Default" w282 {
          tunnel: w285 -> [_ w305]
          tunnel: [enum16{"cnfg", "inc", "mph", "err", "RSET"}."RSET" w305] -> w283
          frame Default {
            w302 = 0.0 ("MPH")
            n118 = local write "ESTOP"(TRUE ("ESTOP")) -> ()
            n119 = local write "MPH 2"(w302) -> ()
            n120 = local write "MPH"(w302) -> ()
          }
          frame -1 {
          }
        }
      }
      frame "Error" {
        n121 = local read "stopping"() -> (w318:bool)
        n122 = Compound Arithmetic op=OR("stop", w318, w317) -> (w320:bool)
        n123 = case shown="True" w320 {
          tunnel: [FALSE TRUE] -> w316
          frame False {
          }
          frame True {
            n124 = local write "stopping"(TRUE ("stopping")) -> ()
          }
        }
      }
    }
  }
  n125 = VISA Close(VISA resource name=w9, error in (no error)=w8) -> (error out=w7:errorcluster)
  n126 = call <vilib>:"DAQmx Clear Task.vi"("task in"=w4, "error in"=w5) -> ("error out"=w3:errorcluster)  [unwired: 13 in]
  n127 = call <vilib>:"Simple Error Handler.vi"("error in (no error)"=w7) -> ()  [unwired: 4 in, 5 out]
  n128 = call <vilib>:"Simple Error Handler.vi"("error in (no error)"=w3) -> ()  [unwired: 4 in, 5 out]
